vi "Factory.vi"(8 "error in (no error)":errorcluster, 11 "File Parser Interface in":refnum<class "File Parser Interface.lvclass">) -> (0 "error out":errorcluster, 3 "File Parser Interface out":refnum<class "File Parser Interface.lvclass">)   [LabVIEW 2018, in "File Parser Interface.lvlib" / "File Parser Interface.lvclass"]
uses:
  File Parser Interface.lvclass
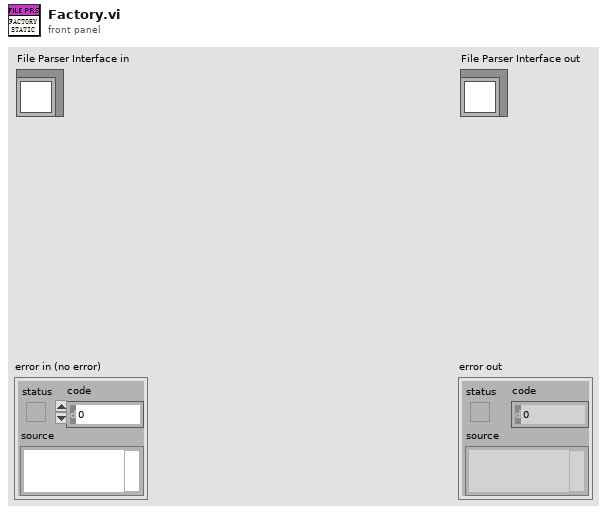
[diagram p1: front panel]
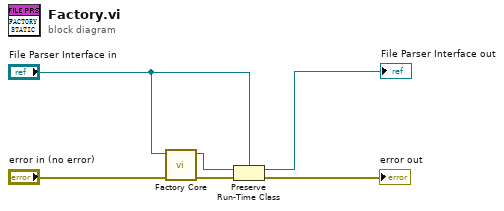
[diagram p0: block diagram]
diagram:
  n1 = call-dynamic "Factory Core.vi"("error in (no error)"="error in (no error)", "File Parser Interface in"="File Parser Interface in") -> ("error out"=w5:errorcluster, "File Parser Interface out"=w3:refnum<class "File Parser Interface.lvclass">)  [unwired: 8 in]
  n2 = Preserve Run-Time Class(object in=w3, error in=w5, 2:"File Parser Interface in") -> (object out=→"File Parser Interface out":refnum<class "File Parser Interface.lvclass">, error out=→"error out":errorcluster)
